vi "Process.vi"(8 "error in (no error)":errorcluster, 10 "Pound in":refnum<class "Pound.lvclass">, 11 "Qbus in":refnum<class "Qbus.lvclass">) -> (0 "error out":errorcluster)   [LabVIEW 2017, in "McsaAnalysisHighRate.lvlib"]
doc: "Calculates high-rate features, such as Percent Full Load Amps and MCSA RMS, from waveforms that the channels in a data group acquire. Subsequent processes can evaluate this feature data to trigger alarms, collect data sets, and perform other operations."
uses:
  <vilib>/addons/InsightCM/Devices/Shared/Mcsa/McsaAnalysisHighRate/McsaAnalysisHighRate.lvlib
  <vilib>/addons/Qbus/Qbus.lvclass
  <vilib>/NI/Software Watchdog/Pound/Pound.lvclass
  <vilib>/addons/InsightCM/Devices/Shared/Mcsa/McsaAnalysisHighRate/controls/Config.ctl
  <vilib>/addons/InsightCM/Devices/Shared/Mcsa/McsaAnalysisHighRate/controls/Group.ctl
  <vilib>/addons/InsightCM/Utilities/Analysis/MCSA/controls/McsaChannel.ctl
  <vilib>/addons/InsightCM/Utilities/Analysis/Shared/controls/Feature.ctl
  <vilib>/addons/InsightCM/Utilities/Analysis/Shared/controls/AmplitudeScale.ctl
  <vilib>/addons/InsightCM/MessageBus/Base/controls/KeyValuePair.ctl
  <vilib>/addons/InsightCM/Utilities/Analysis/MCSA/controls/McsaMotor.ctl
  <vilib>/NI/Software Watchdog/Watchdog/Watchdog.lvclass
  <vilib>/addons/InsightCM/Devices/Shared/Common/DataFlow/DataFlow.lvlib
  <vilib>/addons/InsightCM/Utilities/Analysis/Shared/AnalysisHelper.lvlib
  <vilib>/addons/InsightCM/Utilities/GlobalConfiguration/GlobalConfiguration.lvlib
  <vilib>/addons/InsightCM/Devices/Shared/Common/DataEventCreator/DataEventCreator.lvlib
  <vilib>/addons/InsightCM/Utilities/Analysis/MCSA/McsaAnalysisFunctions.lvlib
  <vilib>/addons/TraceLogger/TraceLogger.lvlib
  <vilib>/addons/InsightCM/Devices/Shared/Mcsa/McsaDataEventCreator/McsaDataEventCreator.lvlib
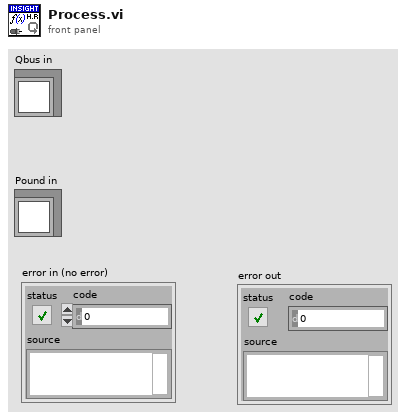
[diagram p1: front panel]
types:
  T1 = typedef "McsaAnalysisHighRate.lvlib/Config.ctl" = cluster{"Device Name":string, "Groups":T2[]}
  T2 = typedef "McsaAnalysisHighRate.lvlib/Group.ctl" = cluster{"Name":string, "Channels":T3[], "Motor Info":T7}
  T3 = typedef "McsaAnalysisFunctions.lvlib/McsaChannel.ctl" = cluster{"Name":string, "Id":string, "Type":string, "Wiring Configuration":string, "Nominal Line Voltage":dbl, "Phase A Channel":string, "Phase B Channel":string, "Phase C Channel":string, "Channel Status":string, "Features":T4[], "Data Valid":bool, "Acq Timestamp":timestamp, "Channel Properties":T6[], "Torque Waveform Unit":string}
  T4 = typedef "AnalysisHelper.lvlib/Feature.ctl" = cluster{"MetricType":string, "TdmsPropName":string, "DisplayName":string, "Unit":string, "Use Volts":bool, "Value":dbl, "Tag Id":string, "Properties":variant, "Amplitude Scale":T5, "valid":bool}
  T5 = typedef "AnalysisHelper.lvlib/AmplitudeScale.ctl" = enum16{"rms", "peak", "pk-pk"}
  T6 = typedef "KeyValuePair.ctl" = cluster{"Key":string, "Value":string}
  T7 = typedef "McsaAnalysisFunctions.lvlib/McsaMotor.ctl" = cluster{"Model":string, "Manufacturer":string, "Serial Number":string, "Horsepower":dbl, "Horsepower Unit":string, "Full Load Speed":dbl, "Synchronous Speed":dbl, "Rated Volts":dbl, "Full Load Amps":dbl, "Frequency":dbl, "Service Factor":dbl, "Efficiency":dbl, "Efficiency @ 75% Load":dbl, "Efficiency @ 50% Load":dbl, "Efficiency @ 25% Load":dbl, "Power Factor":dbl, "VoltageBus":string, "VoltageBus ID":string, "Stator Resistance":dbl, "Estimate Stator Resistance":bool}
  T8 = typedef "DataEventCreator.lvlib/RegisterTrendPoints.ctl" = cluster{"DataGroup":string, "Trends":T9[]}
  T9 = typedef "DataEventCreator.lvlib/Registry_Trend.ctl" = cluster{"TrendPointId":string, "DataSetName":string, "HighRate":bool, "Always Send":bool}
  T10 = typedef "DataFlow.lvlib/Data.ctl" = cluster{"DataGroup":string, "Waveforms":T11, "Map":T12, "Type":T13}
  T11 = typedef "wfmSGL_DVR.ctl" = refnum<data-value>
  T12 = typedef "PointValueMap.lvlib/PointMap.ctl" = refnum<data-value>
  T13 = typedef "DataFlow.lvlib/Type.ctl" = enum16{"High Rate", "Low Rate", "Burst Mode"}
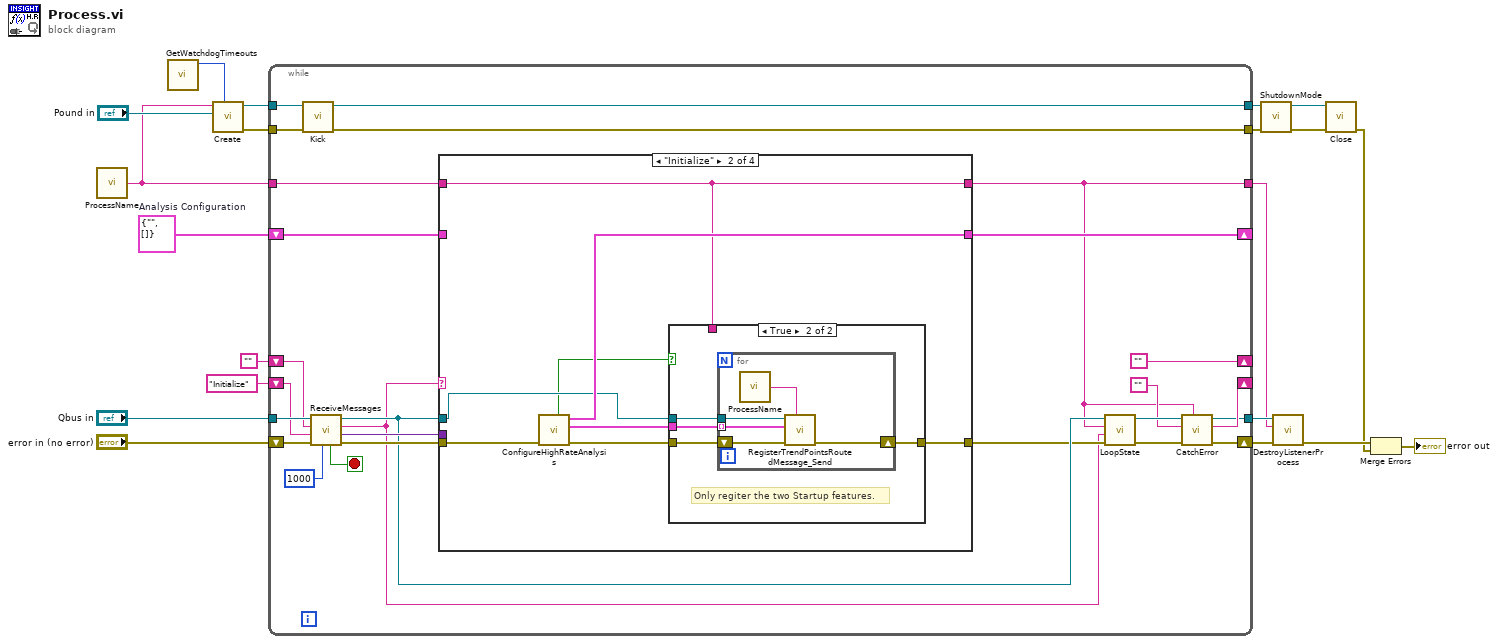
[diagram p0: block diagram]
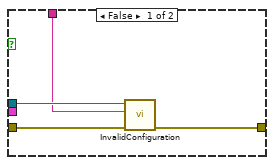
[diagram p3: hidden frame]
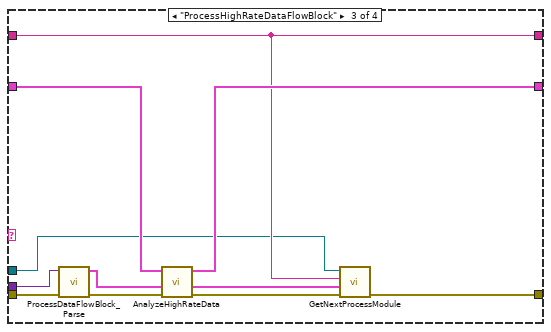
[diagram p4: hidden frame]
diagram:
  w9 = T1 {"Device Name"="", "Groups"=[]}  # Analysis Configuration
  n1 = call <vilib>:"ProcessName.vi"() -> ("ProcessName"=w1:string)  [unwired: 5 in]
  n2 = call <vilib>:"GetWatchdogTimeouts.vi"() -> ("software timeout"=w2:u32)  [unwired: 10 in, 1 out]
  n3 = call <vilib>:"Create.vi"("Execution Timeout (ms)"=w2, "Pound"="Pound in", "Name"=w1) -> ("error out"=w10:errorcluster, "Watchdog"=w11:refnum<data-value>)  [unwired: 7 in]
  n4 = while {
    shift-right: [""] -> _
    shift-left: "" -> [w40]
    shift-right: [w46] -> _
    shift-left: w9 -> [w45]
    shift-right: [w27] -> _
    shift-left: "Initialize" ("MsgName") -> [w38]
    tunnel: w1 -> [w33]
    tunnel: [w26] -> w16
    tunnel: [w24] -> w15
    tunnel: "Qbus in" -> [w43]
    tunnel: [w37] -> w13
    tunnel: [w36] -> w12
    tunnel: w11 -> [w35]
    tunnel: w10 -> [w34]
    shift-right: [w25] -> w17
    shift-left: "error in (no error)" -> [w39]
    stop <- w22 stop-if-true
    n5 = call <vilib>:"Kick.vi"("error in (no error)"=w34, "Watchdog"=w35) -> ("error out"=w37:errorcluster, "Watchdog"=w36:refnum<data-value>)  [unwired: 8 in]
    n6 = call <vilib>:"ReceiveMessages.vi"("Timeout(100)"=1000, "error in (no error)"=w39, "Priority Action"=w38, "Default Action"=w40, "Qbus in"=w43) -> ("error out"=w41:errorcluster, "MsgValue"=w42:variant, "Action"=w23:string, "Qbus out"=w32:refnum<class "Qbus.lvclass">, "Exit"=w22:bool)  [unwired: 2 in]
    n7 = case shown="\"Initialize\"" w23 {
      tunnel: w41 -> [w49 w53 w79 w83]
      tunnel: [w49 w52 w74 w83] -> w31
      tunnel: w42 -> [_ _ w78 _]
      tunnel: [w48 w57 w80 w82] -> w46
      tunnel: w45 -> [w48 _ w81 w82]
      tunnel: w32 -> [_ w56 w73 _]
      tunnel: [w47 w50 w75 w84] -> w24
      tunnel: w33 -> [w47 w50 w75 w84]
      frame Default {
      }
      frame "Initialize" {
        n8 = call <vilib>:"ConfigureHighRateAnalysis.vi"("error in (no error)"=w53) -> ("error out"=w54:errorcluster, "register startup trends"=w55:T8[], "analysis config"=w57:T1, "all config found?"=w51:bool)  [unwired: 7 in]
        n9 = case shown="True" w51 {
          tunnel: w56 -> [w61 w65]
          tunnel: w55 -> [_ w64]
          tunnel: w54 -> [w60 w63]
          tunnel: [w59 w62] -> w52
          tunnel: w50 -> [w58 _]
          frame False {
            n10 = call <vilib>:"InvalidConfiguration.vi"("error in (no error)"=w60, "description"=w58, "Qbus in"=w61) -> ("error out"=w59:errorcluster)  [unwired: 7 in, 1 out]
          }
          frame True {
            # "Only regiter the two Startup features."
            n11 = for {
              tunnel: w64 -> [w70] mode=indexing
              shift-right: [w68] -> w62
              shift-left: w63 -> [w69]
              tunnel: w65 -> [w67]
              n12 = call <vilib>:"ProcessName.vi"() -> ("process name"=w66:string)  [unwired: 5 in]
              n13 = call <vilib>:"RegisterTrendPointsRoutedMessage_Send.vi"("data event creator process name"=w66, "error in (no error)"=w69, "register trend"=w70, "Qbus in"=w67) -> ("error out"=w68:errorcluster)  [unwired: 6 in, 1 out]
            }
          }
        }
      }
      frame "ProcessHighRateDataFlowBlock" {
        n14 = call <vilib>:"ProcessDataFlowBlock_Parse.vi"("error in (no error)"=w79, "body"=w78) -> ("error out"=w72:errorcluster, "data"=w76:T10)  [unwired: 8 in]
        n15 = call <vilib>:"AnalyzeHighRateData.vi"("error in (no error)"=w72, "data in"=w76, "Analysis Configuration In"=w81) -> ("error out"=w71:errorcluster, "data out"=w77:T10, "Analysis Configuration Out"=w80:T1)  [unwired: 6 in]
        n16 = call <vilib>:"GetNextProcessModule.vi"("error in (no error)"=w71, "data"=w77, "source"=w75, "Qbus in"=w73) -> ("error out"=w74:errorcluster)  [unwired: 6 in, 1 out]
      }
      frame "Exit" {
      }
    }
    n17 = call <vilib>:"LoopState.vi"("error in (no error)"=w31, "loop action"=w23, "process name"=w24, "Qbus in"=w32) -> ("error out"=w28:errorcluster, "Qbus out"=w30:refnum<class "Qbus.lvclass">)  [unwired: 6 in]
    n18 = call <vilib>:"CatchError.vi"("source"=w24, "error in (no error)"=w28, "next action in"="", "Qbus in"=w30) -> ("error out"=w25:errorcluster, "next action out"=w27:string, "Qbus out"=w26:refnum<class "Qbus.lvclass">)  [unwired: 5 in]
  }
  n19 = call <vilib>:"ShutdownMode.vi"("error in (no error)"=w13, "Watchdog"=w12) -> ("error out"=w18:errorcluster, "Watchdog"=w19:refnum<data-value>)  [unwired: 8 in]
  n20 = call <vilib>:"DestroyListenerProcess.vi"("error in (no error)"=w17, "process name"=w15, "Qbus in"=w16) -> ("error in (no error)"=w8:errorcluster)  [unwired: 7 in, 1 out]
  n21 = call <vilib>:"Close.vi"("error in (no error)"=w18, "Watchdog"=w19) -> ("error out"=w7:errorcluster)  [unwired: 9 in]
  n22 = Merge Errors(w8, w7) -> (→"error out":errorcluster)
